vi "Write Interlock_Enable.vi"(8 "error in":errorcluster, 10 "INTLK_Enable":bool, 11 "Acopian in":refnum<class "Acopian.lvclass">) -> (0 "error out":errorcluster, 3 "Acopian out":refnum<class "Acopian.lvclass">)   [LabVIEW 2019, in "Acopian.lvlib" / "Acopian.lvclass"]
uses:
  Library/Acopian.lvclass
  C:/Users/Public/Documents/Development/builds/Instruments/Instruments.lvlibp/Library/Instruments.lvclass
  builds/Instruments/Instruments.lvlibp/Accessors/Generate Warning.vi
  builds/Instruments/PowerSupply.lvlibp/Library/PowerSupply.lvclass
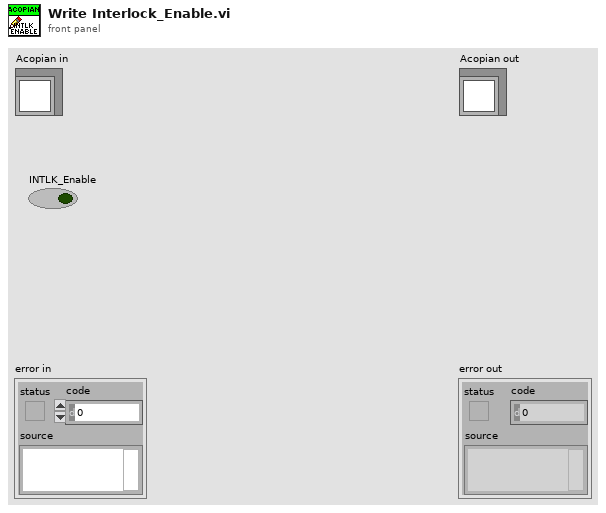
[diagram p1: front panel]
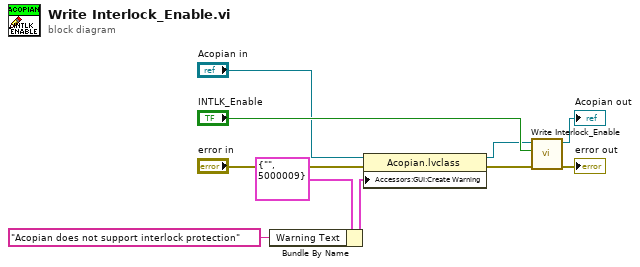
[diagram p0: block diagram]
diagram:
  n1 = Bundle By Name(cluster=cluster{"Warning Text":string, "code":i32} {"Warning Text"="", "code"=5000009} ("Instrument:GUI:Create Warning"), "Warning Text"="Acopian does not support interlock protection") -> (w2:cluster{"Warning Text":string, "code":i32})
  n2 = property class="Acopian.lvclass"(reference="Acopian in", error in="error in", "Accessors:GUI:Create Warning"=w2) -> (reference out=w4:refnum<class "Acopian.lvclass">, error out=w6:errorcluster)
  n3 = call-parent "Write Interlock_Enable.vi"("error in"=w6, "INTLK_Enable"="INTLK_Enable", "PowerSupply in"=w4) -> ("error out"=→"error out":errorcluster, "PowerSupply out"=→"Acopian out":refnum<class "Acopian.lvclass">)  [unwired: 7 in]
